vi "Demultiplexer-Host.vi"() -> ()   [LabVIEW 2012]
uses:
  <vilib>/rvi/interface/nirviOpenFPGA/nirviOpenFPGA.xnode
  <vilib>/rvi/interface/nirviReadWriteControl/nirviReadWriteControl.xnode
  <vilib>/Utility/error.llb/Error Cluster From Error Code.vi
  <vilib>/rvi/interface/Simulation/niFpgaSimulationCallBeginRW.vi
  <vilib>/rvi/errors/niLvFpgaAdjustHostInterfaceError.vi
  NiFpgaLv.dll
  <vilib>/rvi/interface/nirviCloseFPGA/nirviCloseFPGA.xnode
  <vilib>/rvi/interface/nirviMethod/nirviMethod.xnode
  <vilib>/FPGAPlugInAG/Dynamic/niLvFpga_ReadFifo_Dynamic.vi
  <vilib>/rvi/errors/niLvFpgaMergeErrorWithErrorCode.vi
  FPGA Bitfiles/Demultiplexer_Laser80VerySimple160_PXIe-7962R.lvbitx
  <vilib>/FPGAPlugInAG/PXIe-7962R/niLvFpga_Open_PXIe-7962R.vi
  <vilib>/rvi/interface/common/dynamic/niFpgaDynamicAddResources.vi
  <vilib>/FPGAPlugInAG/Dynamic/niLvFpga_Close_Dynamic.vi
panel:
  out "ToHost FIFO Overflow A1Ch2":bool
  out "ToHostCh1Raw FIFO Overflow":bool
  out "ToHostArea1LaserRaw FIFO Overflow":bool
  out "ToHostAreas FIFO overflow":bool
  out "Ch1 raw":i16[](graph)
  in  "Display length":i32=200
  out "Laser raw":i16[](graph)
  out "Regions":i16[](graph)
  out "Calculated laser pulses per pixel":dbl
  out "Pixel time (µs)":dbl
  out "Acquired samples":u32
  in  "Quit":bool
  out "Interloop FIFO overflow":bool
  out "Interloop FIFO timeout":bool
  in  "Samples per pixel A2":u16=10000
  in  "Samples per pixel A1":u16=10000
  in  "Clock Freq (Hz)":dbl=500000000.0 format="%#_6p"
  in  "error in":errorcluster
  # "NI 6587 I/O Module Configuration"
  # "FPGA Diagnostics"
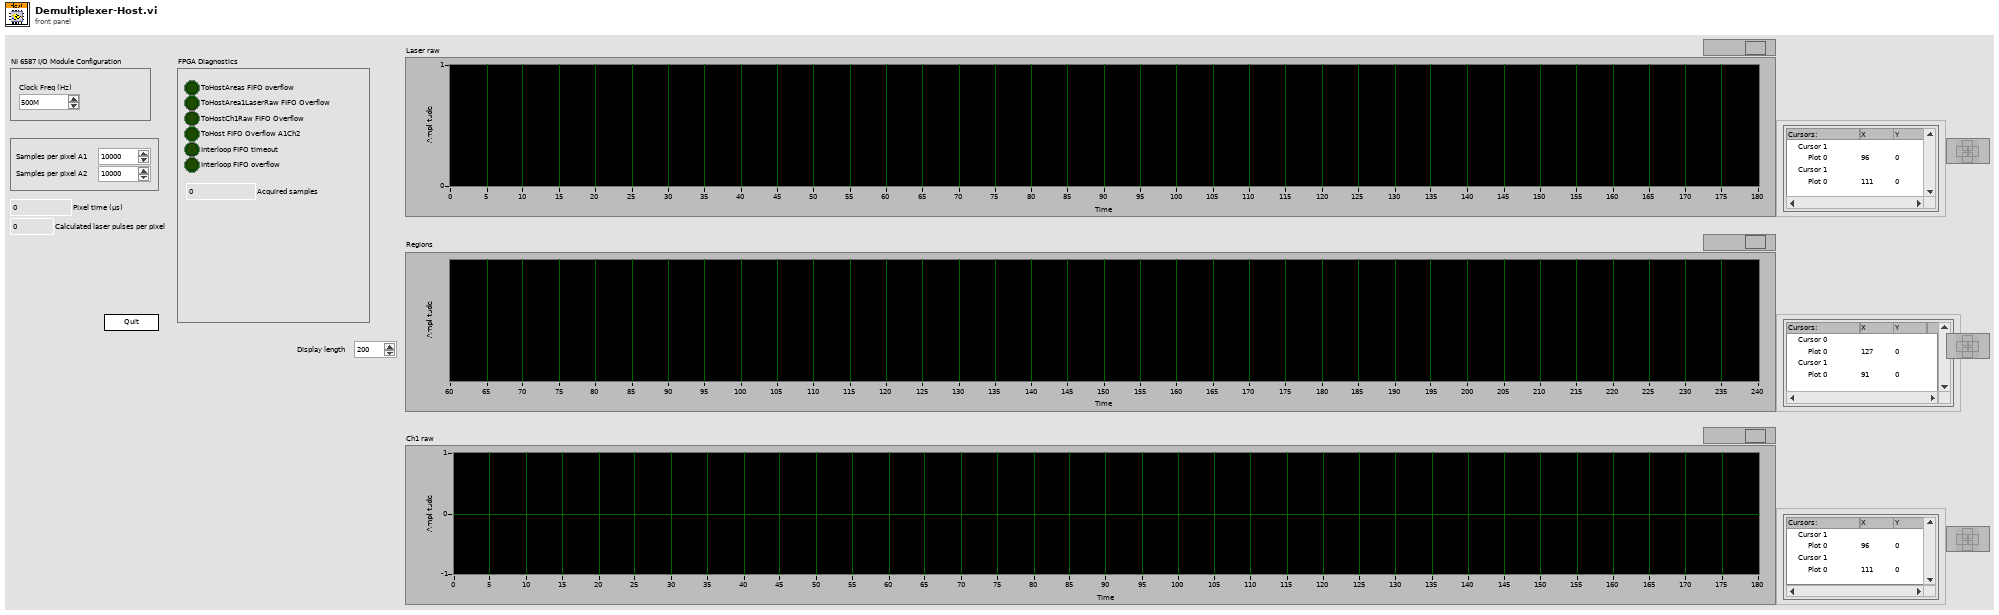
[diagram p1: front panel]
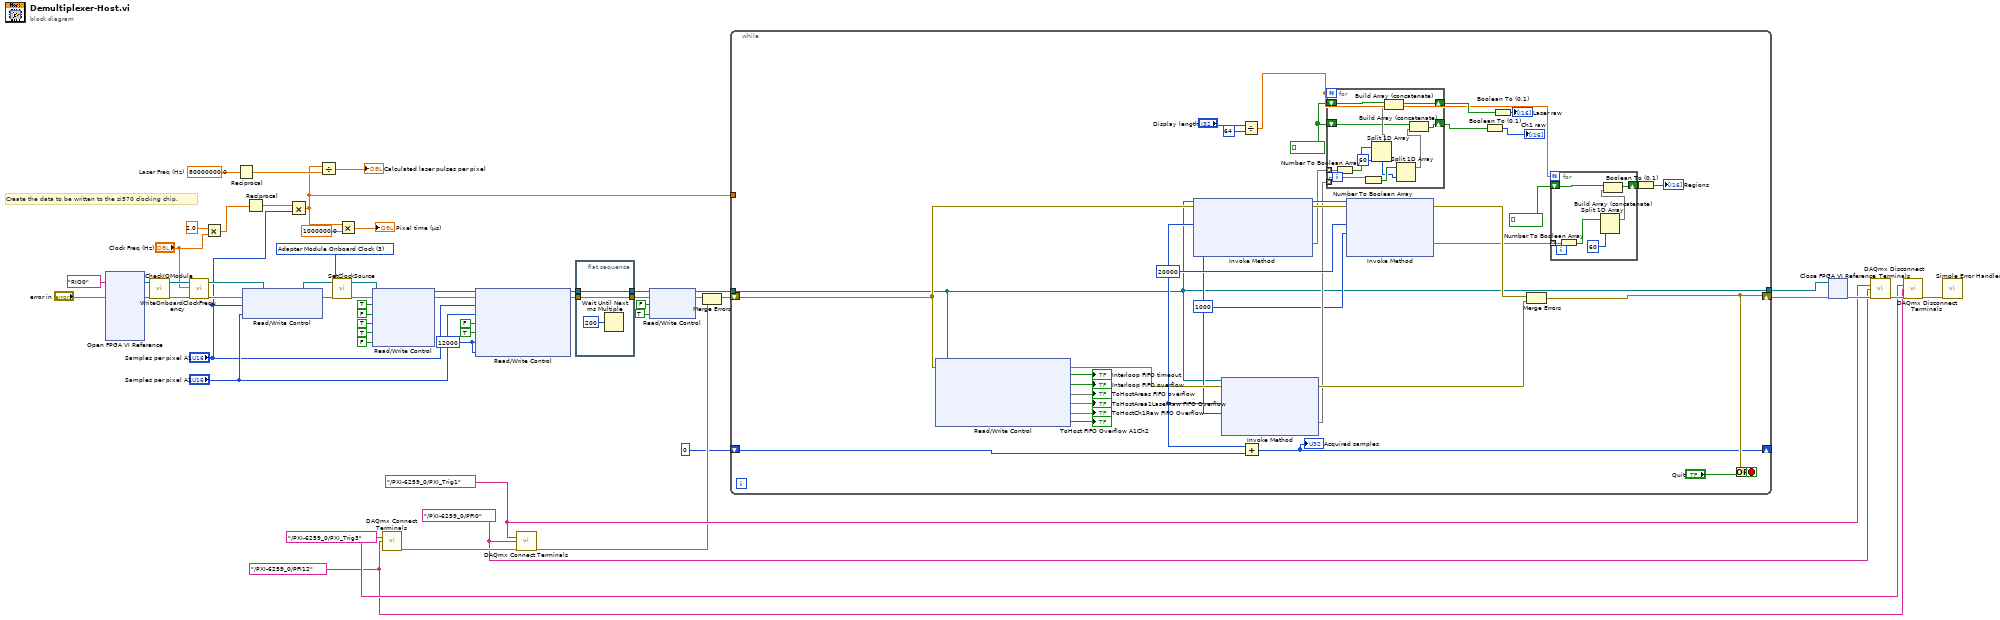
[diagram p0: block diagram]
diagram:
  w1 = u32 12000 ("Switch for")
  w21 = 80000000.0  # Laser Freq (Hz)
  w31 = tag "/PXI-6259_0/PFI0" ("destination terminal")
  w32 = tag "/PXI-6259_0/PXI_Trig1" ("source terminal")
  w29 = tag "/PXI-6259_0/PFI12" ("destination terminal")
  w30 = tag "/PXI-6259_0/PXI_Trig3" ("source terminal")
  w50 = u8 3 items=["Tristate"=0, "Sync Clock (PXIe only)"=2, "Adapter Module Onboard Clock"=3, "Strobe from Crosspoint Switch"=4, "Strobe Bypass"=5] ("Clock Source")
  # "Create the data to be written to the si570 clocking chip."
  n1 = xnode "Open FPGA VI Reference"("error in"="error in", "resource name"=tag "RIO0") -> ("FPGA VI Reference Out"=w53:refnum<k20>, "error out"=w54:errorcluster)
  n2 = call "CheckIOModule.vi"("error in (no error)"=w54, "FPGA VI Reference In"=w53) -> ("error out"=w52:errorcluster, "FPGA VI Reference Out"=w51:refnum<k20>)  [unwired: 8 in]
  n3 = call "WriteOnboardClockFrequency.vi"("error in (no error)"=w52, "Onboard clock frequency"="Clock Freq (Hz)", "FPGA VI Reference In"=w51) -> ("error out"=w48:errorcluster, "FPGA VI Reference Out"=w49:refnum<k20>)  [unwired: 7 in]
  n4 = Multiply(x=2.0, y="Clock Freq (Hz)") -> (x*y=w16:dbl)
  n5 = Reciprocal(x=w21) -> (1/x=w20:dbl)
  n6 = xnode "Read/Write Control"("FPGA VI Reference In"=w49, "error in"=w48, "Samples per pixel A1"="Samples per pixel A1", "Samples per pixel A2"="Samples per pixel A2") -> ("FPGA VI Reference Out"=w46:refnum<k20>, "error out"=w47:errorcluster)
  n7 = Reciprocal(x=w16) -> (1/x=w23:dbl)
  n8 = Multiply(x=w23, y="Samples per pixel A1") -> (x*y=w15:dbl)
  n9 = Divide(x=w15, y=w20) -> (x/y=→"Calculated laser pulses per pixel":dbl)
  n10 = call "SetClockSource.vi"("error in (no error)"=w47, "Clock Source"=w50, "FPGA VI Reference In"=w46) -> ("error out"=w44:errorcluster, "FPGA VI Reference Out"=w45:refnum<k20>)  [unwired: 7 in]
  n11 = Multiply(x=w15, y=1000000.0) -> (x*y=→"Pixel time (µs)":dbl)
  n12 = xnode "Read/Write Control"("FPGA VI Reference In"=w45, "error in"=w44, "Commit"=TRUE, "Acq_Reset"=FALSE, "Acq_Reset"=TRUE, "Acq_Reset"=TRUE, "Wait for trigger"=FALSE) -> ("FPGA VI Reference Out"=w12:refnum<k20>, "error out"=w38:errorcluster)
  n13 = call <vilib>:"DAQmx Connect Terminals.vi"("source terminal"=w30, "destination terminal"=w29) -> ("error out"=w36:errorcluster)  [unwired: 13 in]
  n14 = xnode "Read/Write Control"("FPGA VI Reference In"=w12, "error in"=w38, "Samples per pixel Acq A1"="Samples per pixel A1", "Samples per pixel Acq A2"="Samples per pixel A2", "Acquire"=FALSE, "Acq_Reset"=TRUE, "Requested pixels A2"=w1, "Requested pixels A1"=w1) -> ("FPGA VI Reference Out"=w6:refnum<k20>, "error out"=w5:errorcluster)
  n15 = call <vilib>:"DAQmx Connect Terminals.vi"("source terminal"=w32, "destination terminal"=w31, "error in"=w36) -> ("error out"=w28:errorcluster)  [unwired: 12 in]
  n16 = flat-sequence {
    tunnel: w6 -> [w59]
    tunnel: w5 -> [w58]
    tunnel: [w59] -> w4
    tunnel: [w58] -> w3
    frame #0 {
      n17 = Wait Until Next ms Multiple(millisecond multiple=u32 200) -> ()  [unwired: 1 out]
    }
  }
  n18 = xnode "Read/Write Control"("FPGA VI Reference In"=w4, "error in"=w3, "Acq_Reset"=FALSE, "Acquire"=TRUE) -> ("FPGA VI Reference Out"=w8:refnum<k20>, "error out"=w9:errorcluster)
  n19 = Merge Errors(w9, w28) -> (w27:errorcluster)
  n20 = while {
    shift-right: [w93] -> w25
    shift-left: w27 -> [w61]
    tunnel: w8 -> [w60]
    shift-right: [w89] -> _
    shift-left: u32 0 ("Acquired samples") -> [w90]
    tunnel: [w60] -> w24
    tunnel: w15 -> [_]
    stop <- w91 stop-if-true
    w62 = 1000 ("Timeout (ms)")
    w70 = bool[] []
    w72 = u32 20000 ("Number of Elements")
    n21 = xnode "Read/Write Control"("FPGA VI Reference In"=w60, "error in"=w61) -> ("error out"=w63:errorcluster, "Interloop FIFO timeout"=→"Interloop FIFO timeout":bool, "Interloop FIFO overflow"=→"Interloop FIFO overflow":bool, "ToHostAreas FIFO Overflow"=→"ToHostAreas FIFO overflow", "ToHostArea1LaserRaw FIFO Overflow"=→"ToHostArea1LaserRaw FIFO Overflow", "ToHostCh1Raw FIFO Overflow"=→"ToHostCh1Raw FIFO Overflow", "ToHost FIFO Overflow A1Ch2"=→"ToHost FIFO Overflow A1Ch2":bool)  [unwired: 1 out]
    n22 = xnode "Invoke Method"("FPGA VI Reference In"=w60, "error in"=w61, "Number of Elements"=w72, "Timeout (ms)"=w62) -> ("FPGA VI Reference Out"=w84:refnum<k20>, "error out"=w85:errorcluster, "Data"=w83:void[])  [unwired: 1 out]
    n23 = xnode "Invoke Method"("FPGA VI Reference In"=w60, "error in"=w63, "Number of Elements"=w72, "Timeout (ms)"=w62) -> ("error out"=w86:errorcluster, "Data"=w71:void[])  [unwired: 2 out]
    n24 = Divide(x="Display length", y=64) -> (x/y=w74:dbl)
    n25 = Add(x=w72, y=w90) -> (x+y=w89:u32)
    "Acquired samples" <- w89
    n26 = for {
      N: w74 -> [_]
      tunnel: w83 -> [w108] mode=indexing
      shift-right: [w110] -> w82
      shift-left: w70 -> [w109]
      tunnel: w71 -> [w105] mode=indexing
      shift-right: [w101] -> w69
      shift-left: w70 -> [w102]
      w103 = 60 ("length")
      n27 = Number To Boolean Array(number=w108) -> (Boolean array=w107:bool[])
      n28 = Number To Boolean Array(number=w105) -> (Boolean array=w104:bool[])
      n29 = Split 1D Array(array=w107, index=w103) -> (first subarray=w106:bool[])  [unwired: 1 out]
      n30 = Build Array (concatenate)(w109, w106) -> (w110:bool[])
      n31 = Split 1D Array(array=w104, index=w103) -> (first subarray=w100:bool[])  [unwired: 1 out]
      n32 = Build Array (concatenate)(w102, w100) -> (w101:bool[])
    }
    n33 = xnode "Invoke Method"("FPGA VI Reference In"=w84, "error in"=w85, "Number of Elements"=w72, "Timeout (ms)"=w62) -> ("error out"=w80:errorcluster, "Data"=w79:void[])  [unwired: 2 out]
    n34 = Boolean To (0,1)(Boolean=w69) -> (0, 1=→"Ch1 raw":i16[])
    n35 = Boolean To (0,1)(Boolean=w82) -> (0, 1=→"Laser raw":i16[])
    n36 = Merge Errors(w80, w86) -> (w93:errorcluster)
    n37 = for {
      N: w74 -> [_]
      tunnel: w79 -> [w97] mode=indexing
      shift-right: [w99] -> w77
      shift-left: bool[] [] -> [w98]
      n38 = Number To Boolean Array(number=w97) -> (Boolean array=w95:bool[])
      n39 = Split 1D Array(array=w95, index=60 ("length")) -> (first subarray=w94:bool[])  [unwired: 1 out]
      n40 = Build Array (concatenate)(w98, w94) -> (w99:bool[])
    }
    n41 = Boolean To (0,1)(Boolean=w77) -> (0, 1=→"Regions":i16[])
    n42 = Or(x=w93, y="Quit") -> (x .or. y?=w91:bool)
  }
  n43 = xnode "Close FPGA VI Reference"("FPGA VI Reference In"=w24, "error in"=w25) -> ("error out"=w34:errorcluster)
  n44 = call <vilib>:"DAQmx Disconnect Terminals.vi"("source terminal"=w32, "destination terminal"=w31, "error in"=w34) -> ("error out"=w35:errorcluster)  [unwired: 12 in]
  n45 = call <vilib>:"DAQmx Disconnect Terminals.vi"("source terminal"=w30, "destination terminal"=w29, "error in"=w35) -> ("error out"=w33:errorcluster)  [unwired: 12 in]
  n46 = call <vilib>:"Simple Error Handler.vi"("error in (no error)"=w33) -> ()  [unwired: 4 in, 5 out]
